vi "SIMPLE_Set_Find_Posi.vi"() -> ()   [LabVIEW 2016]
uses:
  <vilib>/Instr/_visa.llb/VISA Set IO Buffer Mask.ctl
  <vilib>/Utility/miscctls.llb/LVPointTypeDef.ctl
  <vilib>/Instr/_visa.llb/VISA Configure Serial Port (Instr).vi
  GEN_2.lvlib
panel:
  in  "Tolerance":dbl
  in  "Expected Theta":dbl
  in  "Set Posi":bool=TRUE
  in  "ID":u8=1 format="%x"
  in  "write":bool
  in  "Baud rate":u32=8000000
  in  "Com port":refnum<visa-resource-name>="COM5"
  in  "stop":bool
  # "Find MT"
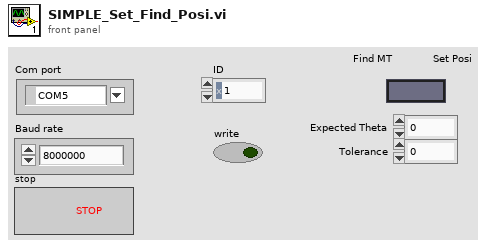
[diagram p1: front panel]
types:
  T1 = typedef "LVPointTypeDef.ctl" = cluster{"Horizontal":i16, "Vertical":i16}
  T2 = typedef "VISA Set IO Buffer Mask.ctl" = u16
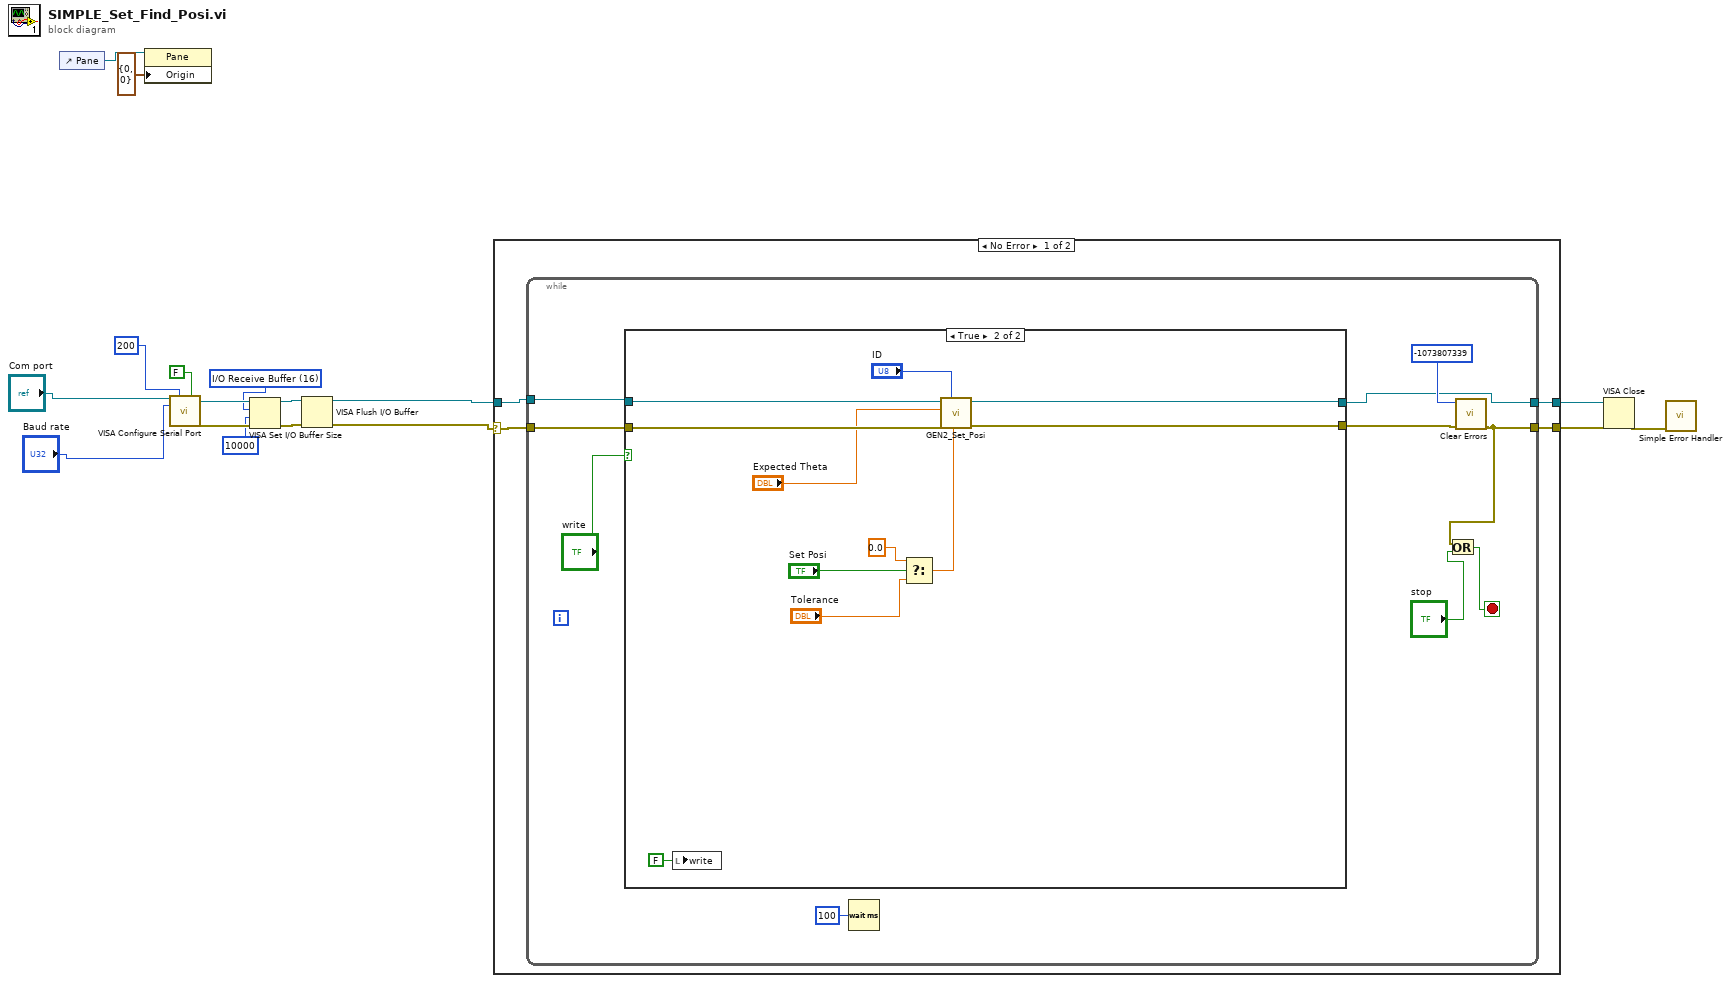
[diagram p0: block diagram]
diagram:
  w9 = T2 16 items=["I/O Receive Buffer"=16, "I/O Transmit Buffer"=32, "I/O Receive and Transmit Buffer"=48] ("Mask")
  n1 = control-ref of="Pane"() -> (w4:refnum<vi>)
  n2 = property class="Pane"(reference=w4, "Origin"=T1 {"Horizontal"=0, "Vertical"=0}) -> ()  [unwired: 1 in, 2 out]
  n3 = call-poly "VISA Configure Serial Port"("VISA resource name"="Com port", "timeout (10sec)"=u32 200, "Enable Termination\nChar (T)"=FALSE ("Enable Termination\nChar (T)"), "baud rate (9600)"="Baud rate") -> ("VISA resource name out"=w10:refnum<visa-resource-name>, "error out"=w13:errorcluster)  [unwired: 10 in]
  n4 = VISA Set I/O Buffer Size(VISA resource name=w10, mask (16)=w9, size (4096)=u32 10000, error in (no error)=w13) -> (VISA resource name out=w11:refnum<visa-resource-name>, error out=w12:errorcluster)
  n5 = VISA Flush I/O Buffer(VISA resource name=w11, error in (no error)=w12) -> (VISA resource name out=w1:refnum<visa-resource-name>, error out=w2:errorcluster)  [unwired: 1 in]
  n6 = case shown="No Error" w2 {
    selector: w2 -> [w18 w45]
    tunnel: [w21 w45] -> w17
    tunnel: w1 -> [w20 w46]
    tunnel: [w19 w46] -> w15
    frame No Error {
      n7 = while {
        tunnel: w20 -> [w27]
        tunnel: w18 -> [w26]
        tunnel: [w24] -> w19
        tunnel: [w25] -> w21
        stop <- w30 stop-if-true
        n8 = case shown="True" "write" {
          tunnel: w26 -> [w33 w40]
          tunnel: w27 -> [w32 w43]
          tunnel: [w32 w42] -> w24
          tunnel: [w33 w41] -> w23
          frame False {
          }
          frame True {
            n9 = local write "write"(FALSE ("write")) -> ()
            n10 = Select(t=0.0, s="Set Posi", f="Tolerance") -> (s? t:f=w36:dbl)
            n11 = call "GEN2_Set_Posi.vi"("Tolerance"=w36, "ID"="ID", "error in (no error)"=w40, "Expected Theta"="Expected Theta", "VISA Refnum in"=w43) -> ("error out"=w41:errorcluster, "VISA Refnum out"=w42:refnum<visa-resource-name>)  [unwired: 5 in]
          }
        }
        n12 = Wait (ms)(milliseconds to wait=u32 100) -> ()  [unwired: 1 out]
        n13 = call <vilib>:"Clear Errors.vi"("error in (no error)"=w23, "specific error code to clear (0: all)"=-1073807339) -> ("error out"=w25:errorcluster)  [unwired: 4 in, 1 out]
        n14 = Or(x=w25, y="stop") -> (x .or. y?=w30:bool)
      }
    }
    frame Error {
    }
  }
  n15 = VISA Close(VISA resource name=w15, error in (no error)=w17) -> (error out=w7:errorcluster)
  n16 = call <vilib>:"Simple Error Handler.vi"("error in (no error)"=w7) -> ()  [unwired: 4 in, 5 out]
